vi "ReadLine.vi"(8 "error in (no error)":errorcluster, 11 "VISA Sesssion In":refnum<visa-resource-name>="ASRL6::INSTR") -> (0 "error out":errorcluster, 2 "Read Line":string, 3 "VISA Sesssion Out":refnum<visa-resource-name>="ASRL6::INSTR")   [LabVIEW 2019]
panel:
  out "output array":u8[](array[numeric])
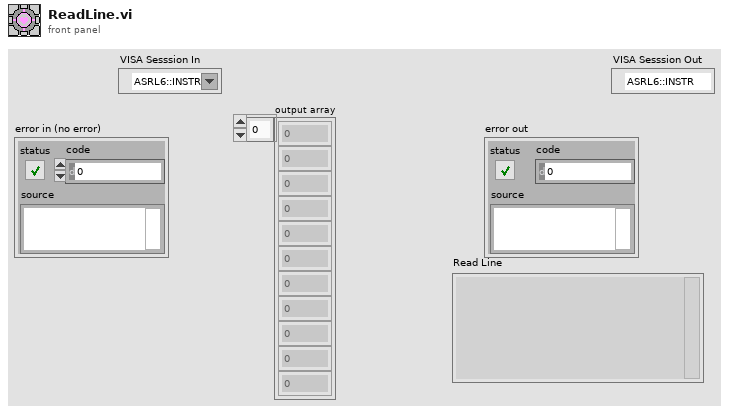
[diagram p1: front panel]
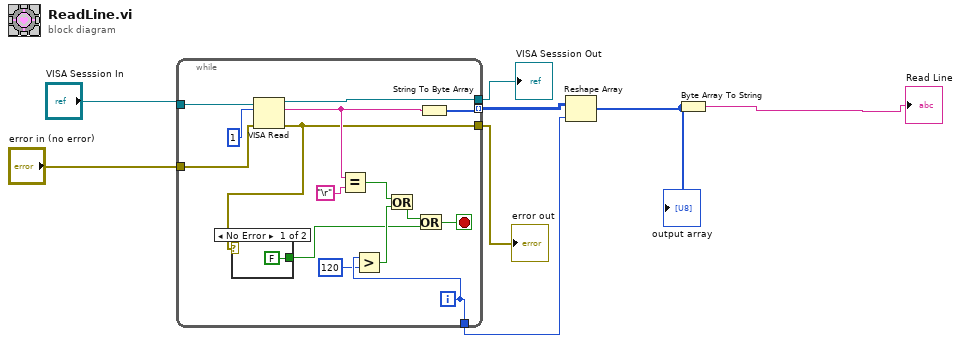
[diagram p0: block diagram]
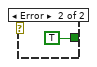
[diagram p2: hidden frame]
diagram:
  n1 = while {
    tunnel: [w18] -> w5 mode=indexing
    tunnel: "VISA Sesssion In" -> [w21]
    tunnel: "error in (no error)" -> [w20]
    tunnel: [w19] -> w1
    tunnel: [w12] -> w7
    tunnel: [w15] -> w4
    i -> [w15]
    stop <- w11 stop-if-true
    n2 = VISA Read(VISA resource name=w21, byte count=u32 1, error in (no error)=w20) -> (VISA resource name out=w19:refnum<visa-resource-name>, read buffer=w17:string, error out=w12:errorcluster)  [unwired: 1 out]
    n3 = case shown="No Error" w12 {
      tunnel: [FALSE TRUE] -> w9
      frame No Error {
      }
      frame Error {
      }
    }
    n4 = Equal?(x=w17, y="\r") -> (x = y?=w16:bool)
    n5 = Greater?(x=w15, y=120) -> (0:w13:bool)
    n6 = Or(x=w16, y=w13) -> (x .or. y?=w10:bool)
    n7 = Or(x=w10, y=w9) -> (x .or. y?=w11:bool)
    n8 = String To Byte Array(string=w17) -> (unsigned byte array=w18:u8[])
  }
  "error out" <- w7
  "VISA Sesssion Out" <- w1
  n9 = Reshape Array(w5, w4) -> (w6:u8[])
  "output array" <- w6
  n10 = Byte Array To String(unsigned byte array=w6) -> (string=→"Read Line":string)
